vi "AguaClara Server.vi"() -> ()   [LabVIEW 2015, in "AguaClara Library.lvlib"]
uses:
  AguaClara Library.lvlib
  Folders.ctl
  Variable cluster.ctl
panel:
  out "total requests":i32
  in  "ADT version":i32
  out "Revision":i32
  in  "SVN Checkout":bool
  out "Loaded CAD":bool
  in  "File Directories":bool
  in  "millisecond multiple":u32=100
  out "stop loops":bool
  in  "stop":bool
  in  "Tab Control":T1(tab)=enum."Test Design"
  out "MathCAD Results":T2
  out "Find-Replace":cluster{"Find":string, "Replace":string}[](array[cluster])
  in  "Load Client Design":i32
  in  "Recreate Design":bool
  out "Date":string
  out "Last Design":i32
  out "init errors":errorcluster caption="error out"
  out "commandline":string
  out "SVN Checkout output":string
  out "design errors":errorcluster
  out "Successful Checkout":bool
  out "Load CAD":errorcluster
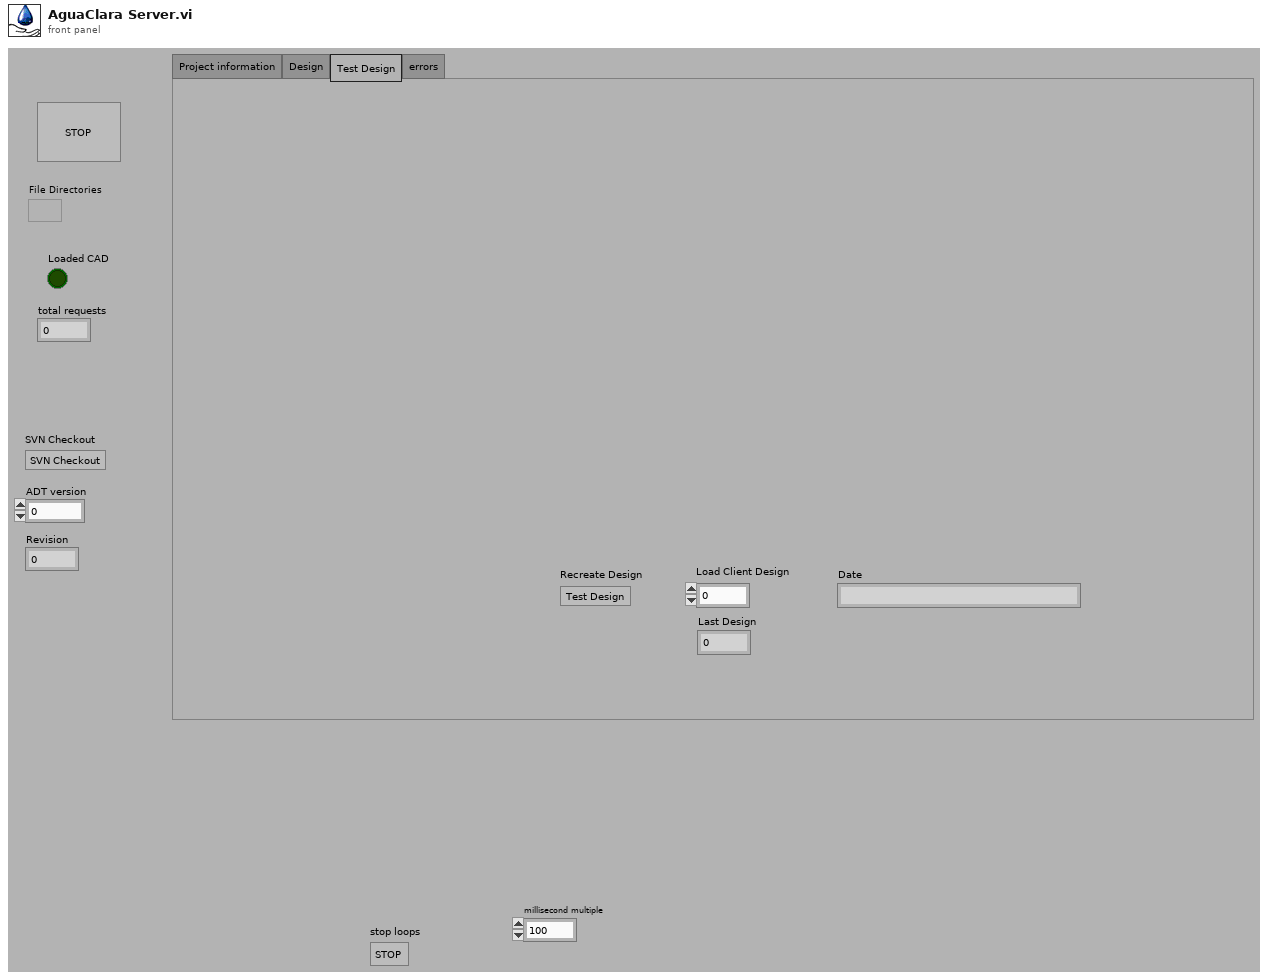
[diagram p1: front panel]
types:
  T1 = enum32{"Project information", "Design", "Test Design", "errors"}
  T2 = typedef "Variable cluster.ctl" = cluster{"Label.Text":string, "Control Type":u32, "Numeric":dbl, "Array":dbl[], "status":bool, "Str Array":string[], "String":string, "unit":string}[]
  T3 = typedef "Folders.ctl" = enum16{"DesignTool", "RequestedDesigns", "CompletedDesigns"}
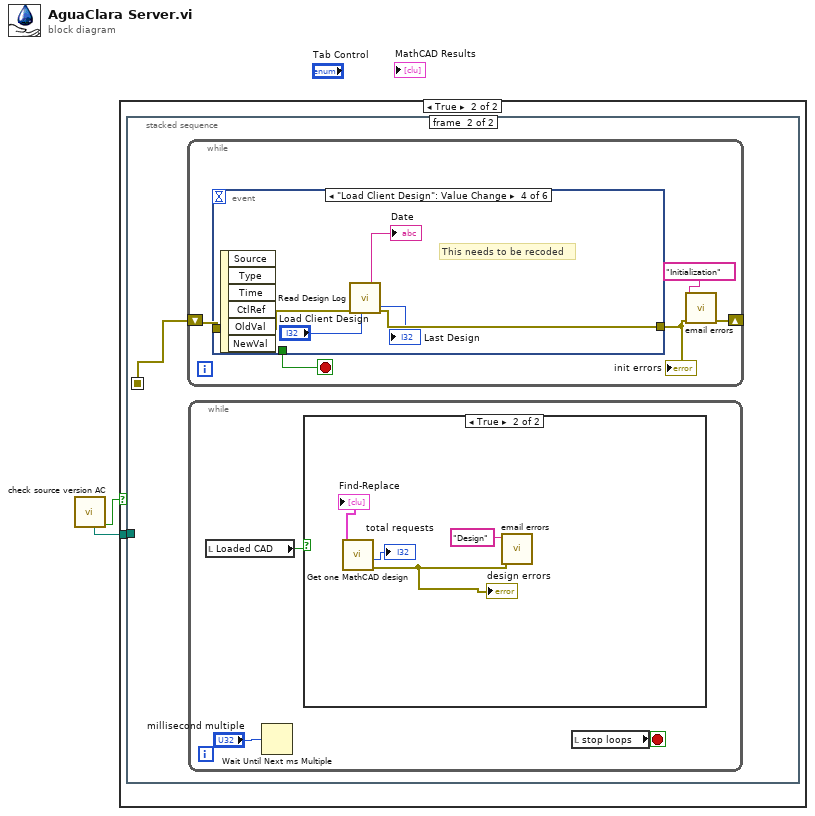
[diagram p0: block diagram]
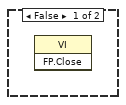
[diagram p2: hidden frame]
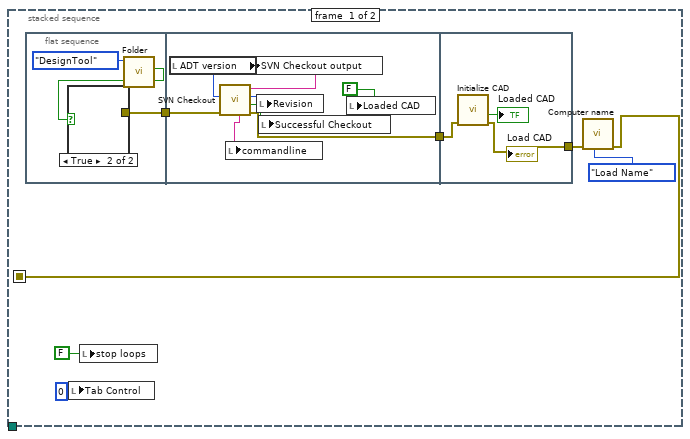
[diagram p3: hidden frame]
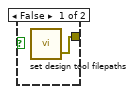
[diagram p4: hidden frame]
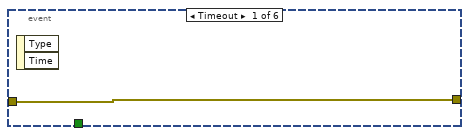
[diagram p6: hidden frame]
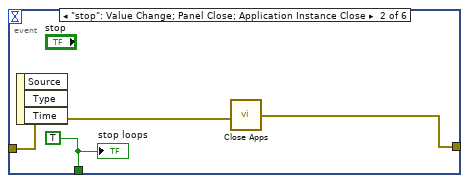
[diagram p7: hidden frame]
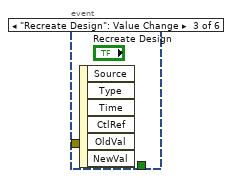
[diagram p8: hidden frame]
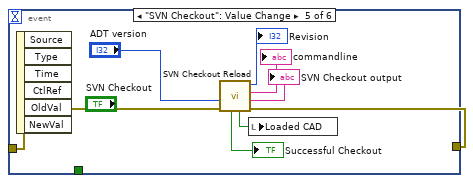
[diagram p9: hidden frame]
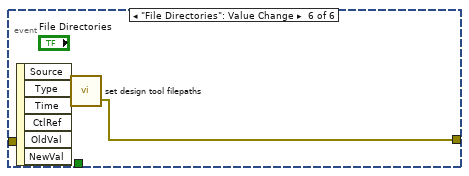
[diagram p10: hidden frame]
diagram:
  n1 = call "check source version AC.vi"() -> ("continue running?"=w2:bool, "Application folder"=w1:path)  [unwired: 3 in, 7 out]
  n2 = case shown="True" w2 {
    tunnel: w1 -> [_ w3]
    frame False {
      n3 = invoke class="VI" method="FP.Close"() -> ()  [unwired: 3 in, 3 out]
    }
    frame True {
      n4 = stacked-sequence {
        seq-local: [w4 _] -> [_ w26]
        tunnel: w3 -> [_ _]
        frame #0 {
          n5 = flat-sequence {
            tunnel: [w11] -> w5
            tunnel: [w18] -> w6
            tunnel: w5 -> [w15]
            tunnel: [w24] -> w7
            tunnel: w6 -> [w23]
            frame #0 {
              n6 = call "Folder.vi"("Folders"=Folders."DesignTool") -> ("found?"=w12:bool)  [unwired: 9 in, 1 out]
              n7 = case shown="True" w12 {
                tunnel: [w14 _] -> w11
                frame False {
                  n8 = call "set design tool filepaths.vi"() -> ("error out"=w14:errorcluster)  [unwired: 2 in, 1 out]
                }
                frame True {
                }
              }
            }
            frame #1 {
              n9 = local read "ADT version"() -> (w21:i32)
              n10 = call "SVN Checkout.vi"("error in (no error)"=w15, "ADT version"=w21) -> ("error out"=w18:errorcluster, "Successful Checkout"=w16:bool, "Revision"=w19:i32, "standard output"=w20:string, "commandline"=w17:string)  [unwired: 5 in]
              n11 = local write "commandline"(w17) -> ()
              n12 = local write "SVN Checkout output"(w20) -> ()
              n13 = local write "Revision"(w19) -> ()
              n14 = local write "Successful Checkout"(w16) -> ()
              n15 = local write "Loaded CAD"(FALSE ("Loaded CAD")) -> ()
            }
            frame #2 {
              n16 = call "Initialize CAD.vi"("error in (no error)"=w23) -> ("error out"=w24:errorcluster, "Success"=→"Loaded CAD":bool)  [unwired: 9 in]
              "Load CAD" <- w24
            }
          }
          n17 = local write "Tab Control"(u8 0 ("Disabled")) -> ()
          n18 = local write "stop loops"(FALSE ("stop loops")) -> ()
          n19 = call "Computer name.vi"("cmd"=enum16{"Load Name", "Read Name"}."Load Name", "error in (no error)"=w7) -> ("error out"=w4:errorcluster)  [unwired: 8 in, 1 out]
        }
        frame #1 {
          n20 = while {
            shift-right: [w36] -> _
            shift-left: w26 -> [w37]
            stop <- w38 stop-if-true
            n21 = event shown="[3] \"Load Client Design\": Value Change" {
              selector: _ -> [_ _ _ _ _ _]
              dyn-events: _ -> [_ _ _ _ _ _]
              timeout: _ -> [_ _ _ _ _ _]
              tunnel: [_ w42 _ _ _ _] -> w38
              tunnel: [w39 w41 _ w46 w54 w56] -> w35
              tunnel: w37 -> [w39 w40 _ w47 w55 _]
              event Timeout {
                n22 = event-data() -> ()  [unwired: 1 in, 2 out]
              }
              event "stop": Value Change; Panel Close; Application Instance Close {
                w42 = TRUE
                n23 = event-data() -> ()  [unwired: 1 in, 3 out]
                n24 = call "Close Apps.vi"("error in"=w40) -> ("error out"=w41:errorcluster)
                "stop loops" <- w42
              }
              event "Recreate Design": Value Change {
                n25 = event-data() -> ()  [unwired: 1 in, 6 out]
              }
              event "Load Client Design": Value Change {
                # "This needs to be recoded"
                n26 = event-data() -> ()  [unwired: 1 in, 6 out]
                n27 = call "Read Design Log.vi"("Design Log Index"="Load Client Design", "error in (no error)"=w47) -> ("error out"=w46:errorcluster, "Last Design"=→"Last Design":i32, "Date"=→"Date":string)  [unwired: 4 in, 3 out]
              }
              event "SVN Checkout": Value Change {
                n28 = event-data() -> ()  [unwired: 1 in, 6 out]
                n29 = call "SVN Checkout Reload.vi"("error in"=w55, "ADT version"="ADT version") -> ("error out"=w54:errorcluster, "SVN Checkout output"=→"SVN Checkout output":string, "commandline"=→"commandline":string, "Revision"=→"Revision":i32, "Success"=w50:bool, "Successful Checkout"=→"Successful Checkout":bool)  [unwired: 4 in]
                n30 = local write "Loaded CAD"(w50) -> ()
              }
              event "File Directories": Value Change {
                n31 = event-data() -> ()  [unwired: 1 in, 6 out]
                n32 = call "set design tool filepaths.vi"() -> ("error out"=w56:errorcluster)  [unwired: 2 in, 1 out]
              }
            }
            "init errors" <- w35
            n33 = call "email errors.vi"("error in (no error)"=w35, "Loop id"="Initialization") -> ("error out (no error)"=w36:errorcluster)  [unwired: 9 in]
          }
          n34 = while {
            stop <- w29 stop-if-true
            n35 = local read "Loaded CAD"() -> (w28:bool)
            n36 = Wait Until Next ms Multiple(millisecond multiple="millisecond multiple") -> ()  [unwired: 1 out]
            n37 = case shown="True" w28 {
              frame False {
              }
              frame True {
                n38 = call "Get one MathCAD design.vi"() -> ("error out"=w33:errorcluster, "Number of Pending Requests"=→"total requests":i32, "Find-Replace"=→"Find-Replace":cluster{"Find":string, "Replace":string}[])  [unwired: 7 in, 2 out]
                "design errors" <- w33
                n39 = call "email errors.vi"("error in (no error)"=w33, "Loop id"="Design") -> ()  [unwired: 9 in, 1 out]
              }
            }
            n40 = local read "stop loops"() -> (w29:bool)
          }
        }
      }
    }
  }
